vi "Name Xbox Inputs.vi"(2 "Axes":dbl[](array[numeric]), 3 "Buttons":bool[](array[boolean])) -> (0 "Named_Joystick":T1, 1 "Named_Buttons":T2)   [LabVIEW 2015]
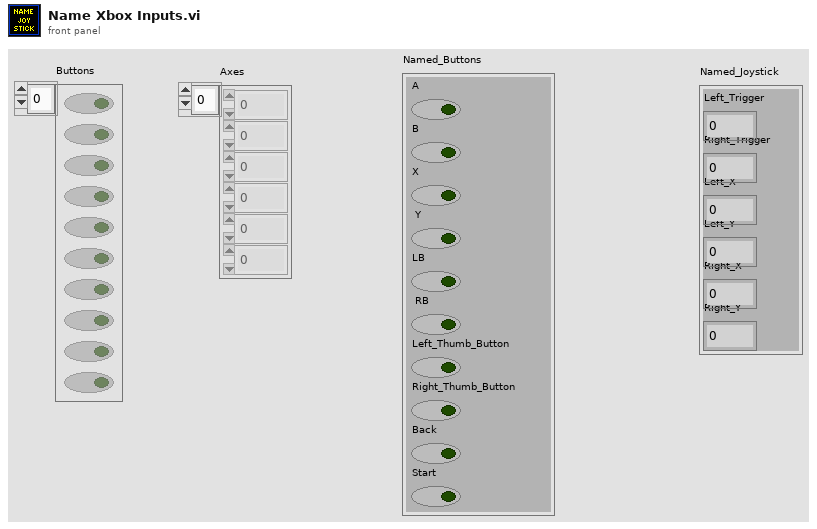
[diagram p1: front panel]
types:
  T1 = cluster{"Left_Trigger":dbl, "Right_Trigger ":dbl, "Left_X":dbl, "Left_Y":dbl, "Right_X":dbl, "Right_Y":dbl}
  T2 = cluster{"A":bool, "B":bool, "X":bool, " Y":bool, "LB":bool, " RB":bool, "Left_Thumb_Button":bool, "Right_Thumb_Button":bool, "Back":bool, "Start":bool}
  T3 = cluster{"Axes[0]":dbl, "Axes[1]":dbl, "Axes[2]":dbl, "Axes[3]":dbl, "Axes[4]":dbl, "Axes[5]":dbl}
  T4 = cluster{"Buttons[0]":bool, "Buttons[1]":bool, "Buttons[2]":bool, "Buttons[3]":bool, "Buttons[4]":bool, "Buttons[5]":bool, "Buttons[6]":bool, "Buttons[7]":bool, "Buttons[8]":bool, "Buttons[9]":bool}
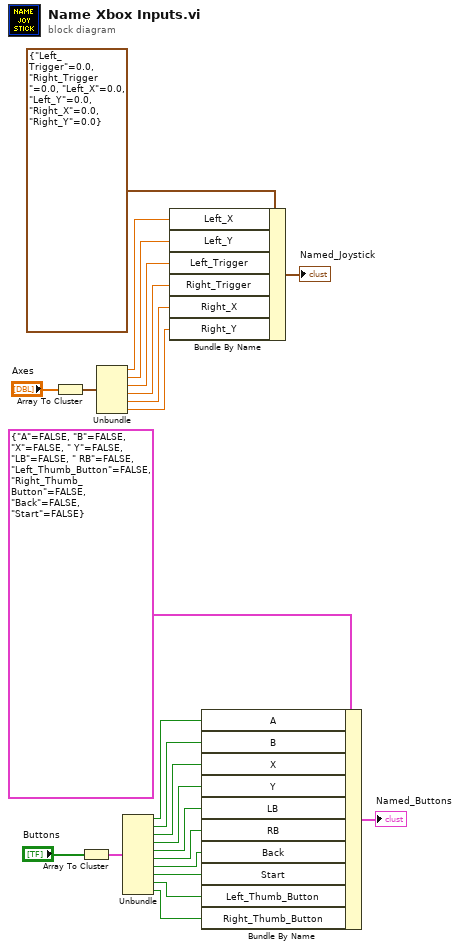
[diagram p0: block diagram]
diagram:
  n1 = Array To Cluster(array="Axes") -> (cluster=w2:T3)
  n2 = Array To Cluster(array="Buttons") -> (cluster=w12:T4)
  n3 = Unbundle(w2) -> ("Axes[0]"=w4:dbl, "Axes[1]"=w5:dbl, "Axes[2]"=w6:dbl, "Axes[3]"=w7:dbl, "Axes[4]"=w8:dbl, "Axes[5]"=w9:dbl)
  n4 = Unbundle(w12) -> ("Buttons[0]"=w15:bool, "Buttons[1]"=w16:bool, "Buttons[2]"=w17:bool, "Buttons[3]"=w18:bool, "Buttons[4]"=w19:bool, "Buttons[5]"=w20:bool, "Buttons[6]"=w21:bool, "Buttons[7]"=w22:bool, "Buttons[8]"=w23:bool, "Buttons[9]"=w11:bool)
  n5 = Bundle By Name(cluster=T1 {"Left_Trigger"=0.0, "Right_Trigger "=0.0, "Left_X"=0.0, "Left_Y"=0.0, "Right_X"=0.0, "Right_Y"=0.0}, "Left_X"=w4, "Left_Y"=w5, "Left_Trigger"=w6, "Right_Trigger"=w7, "Right_X"=w8, "Right_Y"=w9) -> (→"Named_Joystick":T1)
  n6 = Bundle By Name(cluster=T2 {"A"=FALSE, "B"=FALSE, "X"=FALSE, " Y"=FALSE, "LB"=FALSE, " RB"=FALSE, "Left_Thumb_Button"=FALSE, "Right_Thumb_Button"=FALSE, "Back"=FALSE, "Start"=FALSE}, "A"=w15, "B"=w16, "X"=w17, "Y"=w18, "LB"=w19, "RB"=w20, "Back"=w21, "Start"=w22, "Left_Thumb_Button"=w23, "Right_Thumb_Button"=w11) -> (→"Named_Buttons":T2)
